vi "SOUR_POW_START.vi"(0 "VISA IN":refnum<visa-resource-name>, 1 "Start Power":i32, 5 "error in":errorcluster, 7 "Channel":i32) -> (14 "VISA Out":refnum<visa-resource-name>, 19 "error out":errorcluster)   [LabVIEW 2018, in "PNA-X.lvlib"]
doc: "SOURce:POWer:START <num>. \nParameters \n<cnum> Any existing channel number. If unspecified, value is set to 1 \n<num> Start power. \nNote: The range of settable power values depends on the PNA model and if \nsource attenuators are installed. To determine the range of values, perform a \nquery using MAX, then MIN, as an argument. (SOUR:POW:ATT:AUTO must \nbe set to ON) Example: SOURce:POWer:STOP? MAX \nActual achievable leveled power depends on frequency. \nExamples SOUR:POW:STOP -15 \nsource2:power:stop -7 \nQuery Syntax SOURce<cnum>:POWer:STOP? \nReturn Type Numeric \nDefault 0 dBm \nLast modified: \n10/18/06 MQQ Added Mode command \n1833\n\nSource:Power:Correction Commands \nControls the source power calibration features of the analyzer. \nClick on a blue keyword to view the command details. \nSee Also \nExample program using these commands. \nTemplate for creating your own Power Meter Driver \nLearn about Source Power Cal \nSynchronizing the PNA and Controller \nSCPI Command Tree \nNote: The SOURce:POWer:CORRection:COLLect:ACQuire command, used to step the PNA and read a \npower meter, cannot be sent over the GPIB unless the power meter is connected to a different GPIB \ninterface. See the alternative methods described in the command details. \nSOURce<cnum>:POWer<port>:CORRection:COLLect:ABORt \n1834\n\n(Write-only) Aborts a source power calibration sweep that is in progress. \nParameters \n<cnum> Any existing channel number. If unspecified, value is set to 1 \n<port> Port number to correct for source power. If unspecified, value is set to 1. \nExamples SOUR:POW:CORR:COLL:ABOR \nsource1:power2:correction:collect:abort \nQuery Syntax Not Applicable \nDefault Not Applicable \nSOURce<cnum>:POWer<port>:CORRection:COLLect[:ACQuire] <char>,<id>[,src] \nNote: With PNA Rev. 6.2, a new \"id\" argument has been added to this command, replacing \nSOUR:POW:CORR:COLL:METH. \n(Write-only) Initiates a source power cal acquisition sweep using the power sensor attached to the \nspecified channel (A or B) on the power meter, or using the specified PNA receiver. \nNote: This command, when used with a power meter, cannot be sent over the GPIB unless the power \nmeter is connected to a different GPIB interface. Use one of the following methods to perform this \ncommand or its equivalent: \nIf present, use the GPIB dedicated controller port. \nConnect the power meter to the PNA using a USB / GPIB interface (Agilent 82357A). \nSCPI programming of the PNA using a LAN Client interface (see example) \nSend SCPI commands through the COM interface using the SCPI String Parser object. \nDirectly control the Power Meter and PNA to step frequency; then acquire and store the Power reading. \n(see example). \nParameters \n<cnum> Any existing channel number. If unspecified, value is set to 1 \n<port> Port number to correct for source power. If unspecified, value is set to 1. \n<char> The following choices are new beginning PNA Rev 6.2. Choose from: \nPMETer - Power Meter is used for all readings. \nPMReceiver - Power meter for the first iteration; then use the reference receiver \nfor remaining readings if necessary (same as \"fast iteration\" box checked on \n1835\n\ndialog box) \nRECeiver - Use PNA measurement receiver for all readings. \nThe following choices are superseded but still supported, in conjunction with \nSOUR:POW:CORR:COLL:METH. \nASENsor - Sensor on power meter channel A \nBSENsor - Sensor on power meter channel B \n<id> String. Not case sensitive. The power sensor or PNA receiver to use for \nmeasuring power. \nFor PMETer or PMRECeiver: select \"ASENSOR\" or \"BSENSOR\". \nFor RECeiver: select a PNA receiver to acquire readings using physical or logical \nreceiver notation. \nFor ASENsor or BSENsor, this argument is NOT required. \n[src] String. (NOT case sensitive). Source port. Optional. Use SOUR:CAT? to \nreturn a list of valid port names. \nWhile this argument can be used to make settings for ALL ports, it is designed \nto access ports that are not simple numbers, such as \"Port 1 Src2\". Otherwise, \nthe <port> argument performs the same function. If both arguments are \nspecified, [src] takes priority. \nExamples SOUR:POW:CORR:COLL PMET 'acquires power meter readings using \nthe A sensor. \nsource1:power2:correction:collect:acquire receiver,\"a1\" \n'acquires source cal readings using the reference receiver for \nport 1. \nQuery Syntax Not Applicable \nDefault Not Applicable"
uses:
  PNA-X.lvlib
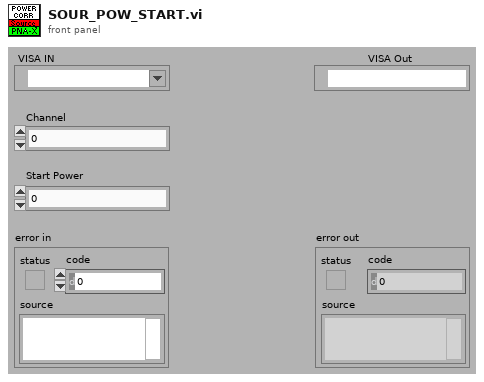
[diagram p1: front panel]
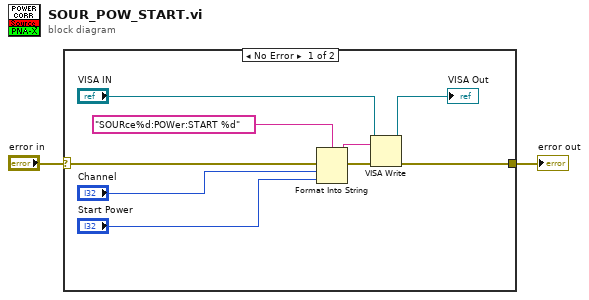
[diagram p0: block diagram]
diagram:
  n1 = case shown="No Error" "error in" {
    selector: "error in" -> [w11 w12]
    tunnel: [w6 w12] -> w1
    frame No Error {
      n2 = Format Into String(format string="SOURce%d:POWer:START %d" ("Cmdline"), error in=w11, "Channel", "Start Power") -> (resulting string=w9:string, error out=w10:errorcluster)  [unwired: 1 in]
      n3 = VISA Write(VISA resource name="VISA IN", write buffer=w9, error in (no error)=w10) -> (VISA resource name out=→"VISA Out":refnum<visa-resource-name>, error out=w6:errorcluster)  [unwired: 1 out]
    }
    frame Error {
    }
  }
  "error out" <- w1
